vi "Intan_mainControlPanel_64chan_ambulatory_v02.vi"() -> ()   [LabVIEW 2017]
panel:
  in  "Experiment Duration (hr)":u16=20
  out "FileSize(MB)":i16
  out "ADC calib":bool
  in  "Config Hardware Filter":bool=TRUE
  in  "ConfigReg [0:7, aPwr]":bool=TRUE
  in  "R_L source":u8(ring)=1 items=["ON-chip", "OFF-chip"]
  in  "Lower cutoff":u8(ring)=12 items=["10 Hz", "7.5 Hz", "5.0 Hz", "3.0 Hz", "2.5 Hz", "2.0 Hz", "1.5 Hz", "1.0 Hz", "0.75 Hz", "0.5 Hz", "0.3 Hz", "0.25 Hz", "0.10 Hz"]
  in  "Upper cutoff":u8(ring)=12 items=["5.0 kHz", "3.0 kHz", "2.5 kHz", "2.0 kHz", "1.5 kHz", "1.0 kHz", "750 Hz", "500 Hz", "300 Hz", "250 Hz", "200 Hz", "150 Hz", "100 Hz"]
  out "DT stream (us)":dbl
  out "ADC_UART ratio":i16
  in  "UART Stream  Rate (Hz)":u16=20
  out "DT samp (us)":dbl
  out "ADC fs (Hz)":dbl
  in  "Desired Fs (Hz)":u16=100
  in  "Save to SD card":bool=TRUE
  in  "SD File Name Suffix\n (2 digits)":string="51"
  out "Serial Port Type":string
  in  "VISA resource name":refnum<visa-resource-name>="COM33"
  in  "Start Data Stream":bool
  out "HeaderFilePath":path
  in  "Save Display Data":bool
  out "Config Result":string
  out "Teensy response":string
  out "Raw data file path":path
  in  "Save Raw Data":bool
  # "Intan-Teensy Bioelectric Module: \nconfigure hardware and serial port \nAmbulatory 64 chan"
  # "Configure all settings, then click run arrow.\n\nWhen config is complete, click the purple\nbutton to start data stream.\n\nSeparate VI will pop open to display signals"
  # "UART streaming"
  # "TODO 01 May 2017 JE\n\nSTATUS: Operational, beta.\n\nSOFTWARE issues:\n\n - Set decimation ratio to ensure Nsamps in display never exceeds chart limit\nor sensible human visibility bound (for now set chart history length = 50000.\nFor typical max sampling rates of 500 Hz in our applications, this still allows up to 100 s\nof data display (ridiculously long).  In practice, could probably increase performance\nby decreasing chart history to something smaller like 20000.\n\n\n- Make bdf style header and write to file (low priority)\n\n -  Stream to main fig window, Present only does this in subVI (IntanStream_Parallel Loops.vi)\n  SOLN: just pop open subVI automatically when called, but pre-set filters (?)\n\nHARDWARE issues: \n\n\nNeed to gracefully recover when data sync is lost. Option to reboot Teensy and recover connection? \nCurrent error checking not working, don' know why.  Software reset tricky to implement:\nhttps://forum.pjrc.com/archive/index.php/t-24304.html\nBest solution for now, unplug then replug power.  This puts Teensy back into initial state.\n\n-Option to stream subset of channels.  This will allow higher data rate for wireless streaming, if desired."
  # "Intan Amp Config"
  # "Hardware Filter Settings"
  # "ADC Sampling"
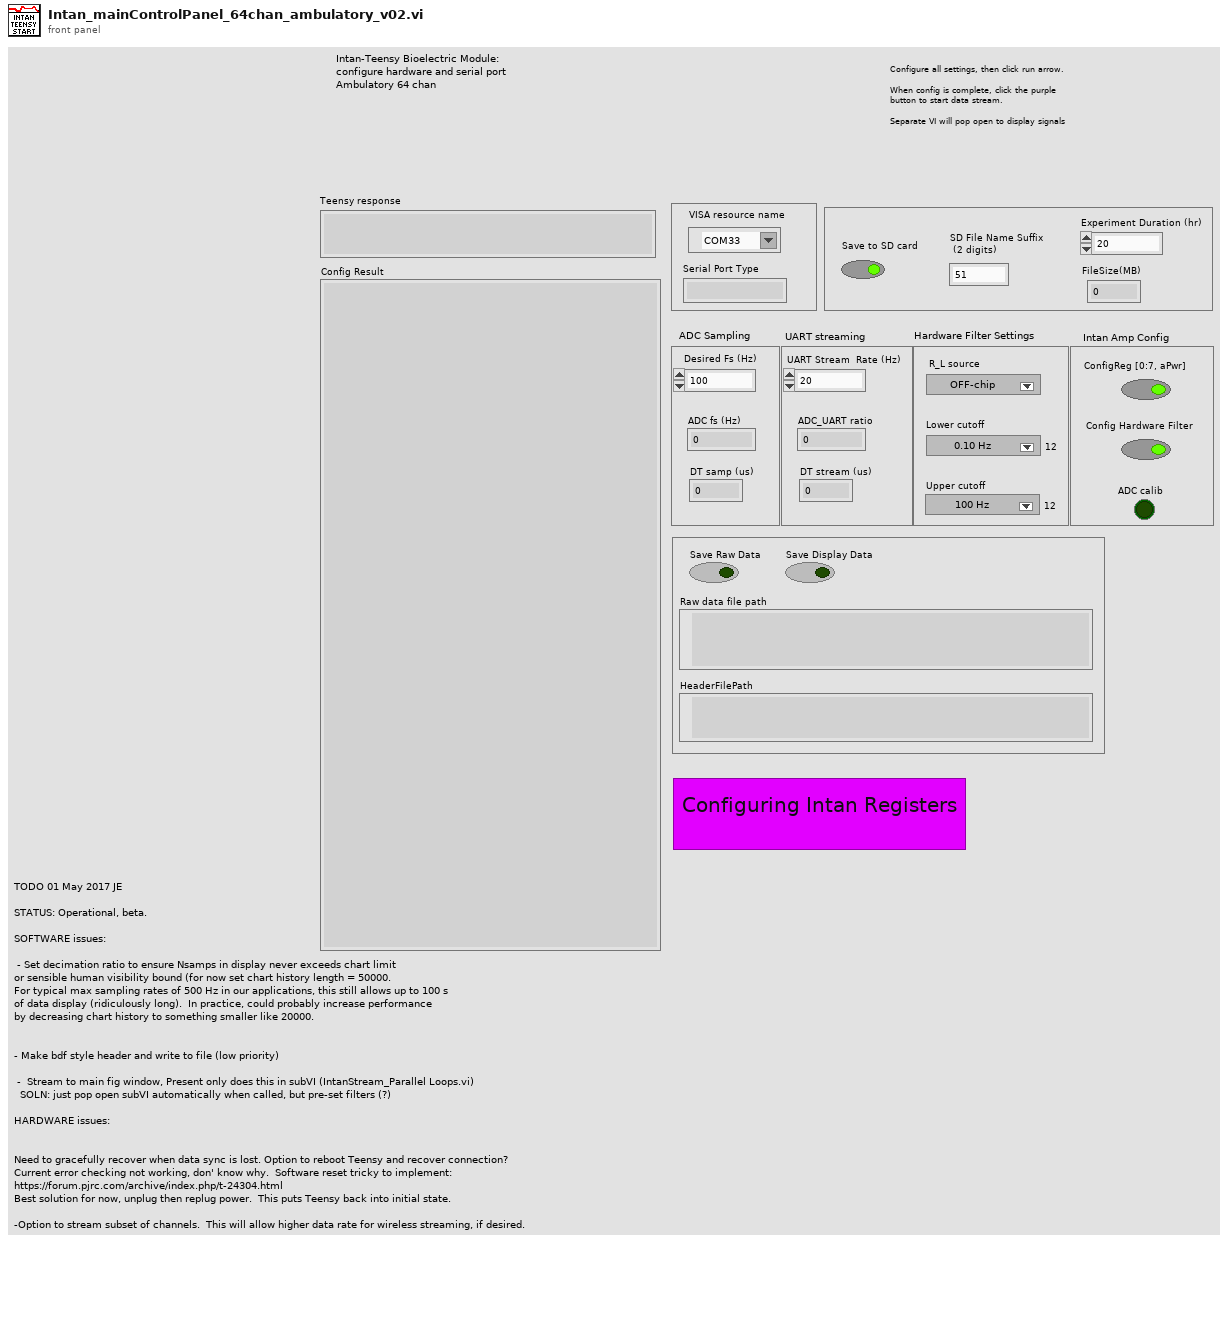
[diagram p1: front panel]
types:
  T1 = enum8{"Enabled", "Disabled", "Disabled and Grayed Out"}
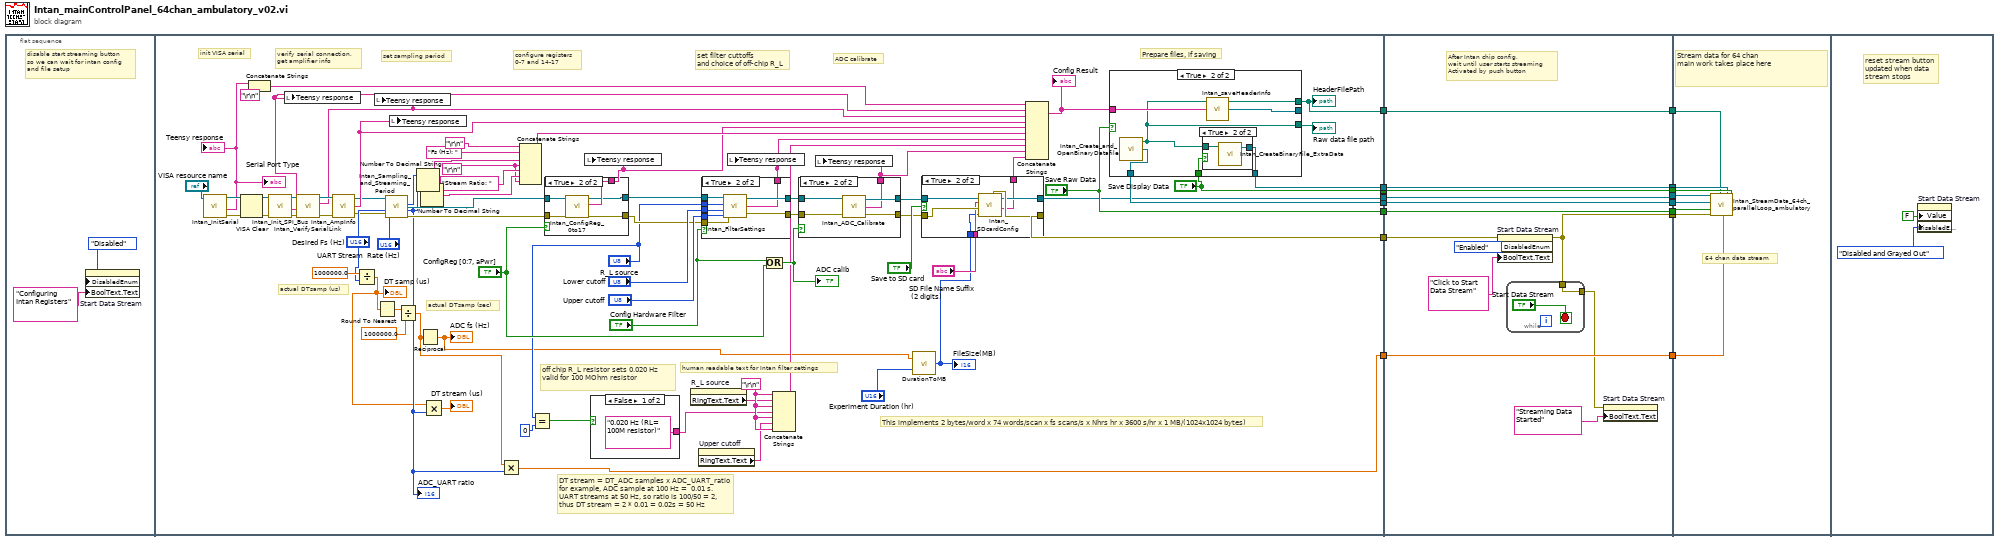
[diagram p0: block diagram]
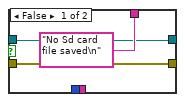
[diagram p2: hidden frame]
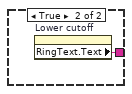
[diagram p3: hidden frame]
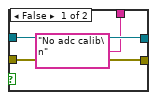
[diagram p4: hidden frame]
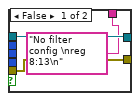
[diagram p5: hidden frame]
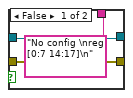
[diagram p6: hidden frame]
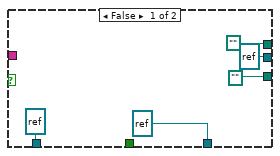
[diagram p7: hidden frame]
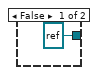
[diagram p8: hidden frame]
diagram:
  n1 = flat-sequence {
    tunnel: [w87] -> w10
    tunnel: [w23] -> w9
    tunnel: [w75] -> w8
    tunnel: ["Save Raw Data"] -> w7
    tunnel: ["Save Display Data"] -> w6
    tunnel: [w35] -> w5
    tunnel: [w57] -> w2
    tunnel: [w33] -> w1
    tunnel: [w153] -> w16
    tunnel: [w159] -> w15
    tunnel: [w158] -> w14
    tunnel: [w157] -> w13
    tunnel: [w156] -> w12
    tunnel: [w155] -> w11
    tunnel: w6 -> [w155]
    tunnel: w7 -> [w156]
    tunnel: w8 -> [w157]
    tunnel: w9 -> [w158]
    tunnel: w10 -> [w159]
    tunnel: w5 -> [w152]
    tunnel: [w151] -> w4
    tunnel: [w150] -> w3
    tunnel: w2 -> [w150]
    tunnel: w1 -> [w151]
    tunnel: w16 -> [w166]
    tunnel: w15 -> [w164]
    tunnel: w14 -> [w169]
    tunnel: w13 -> [w167]
    tunnel: w12 -> [w165]
    tunnel: w11 -> [w168]
    tunnel: w4 -> [w163]
    tunnel: w3 -> [w162]
    frame #0 {
      # "disable start streaming button\nso we can wait for intan config\nand file setup"
      n2 = property on="Start Data Stream" class="Bool (strict)"("DisabledEnum"=T1."Disabled" ("Disabled"), "BoolText.Text"="Configuring Intan Registers" ("Boolean Text.Text")) -> ()  [unwired: 2 in, 2 out]
    }
    frame #1 {
      w52 = "\r\n"
      w26 = "\r\n"
      # "This implements 2 bytes/word x 74 words/scan x fs scans/s x Nhrs hr x 3600 s/hr x 1 MB/(1024x1024 bytes)"
      # "DT stream = DT_ADC samples x ADC_UART_ratio\nfor example, ADC sample at 100 Hz =  0.01 s.\nUART streams at 50 Hz, so ratio is 100/50 = 2,\nthus DT stream = 2 * 0.01 = 0.02s = 50 Hz"
      # "off chip R_L resistor sets 0.020 Hz \nvalid for 100 MOhm resistor"
      # "human readable text for Intan filter settings"
      # "Prepare files, if saving"
      # "ADC calibrate"
      # "set filter cuttoffs \nand choice of off-chip R_L"
      # "configure registers\n0-7 and 14-17"
      # "set sampling period"
      # "verify serial connection,\nget amplifier info"
      # "init VISA serial"
      # "actual DTsamp (sec)"
      # "actual DTsamp (us)"
      n3 = call "Intan_InitSerial.vi"("VISA resource name"="VISA resource name") -> ("VISA resource name out"=w56:refnum<visa-resource-name>, "Text response"=w54:string, "error out"=w86:errorcluster)  [unwired: 3 in]
      "Teensy response" <- w54
      "Serial Port Type" <- w54
      n4 = VISA Clear(VISA resource name=w56, error in (no error)=w86) -> (VISA resource name out=w43:refnum<visa-resource-name>, error out=w42:errorcluster)
      n5 = Concatenate Strings(w54, "\r\n") -> (w39:string)
      n6 = call "Intan_Init_SPI_Bus.vi"("error in"=w42, "VISA resource name"=w43) -> ("error out"=w41:errorcluster, "Text response"=w38:string, "VISA resource name out"=w40:refnum<visa-resource-name>)  [unwired: 3 in]
      n7 = local write "Teensy response"(w38) -> ()
      n8 = call "Intan_VerifySerialLink.vi"("error in"=w41, "VISA resource name"=w40) -> ("error out"=w88:errorcluster, "Text response"=w84:string, "VISA resource name out"=w89:refnum<visa-resource-name>)  [unwired: 7 in]
      n9 = call "Intan_AmpInfo.vi"("error in"=w88, "VISA resource name"=w89) -> ("error out"=w71:errorcluster, "Text response"=w85:string, "VISA resource name out"=w72:refnum<visa-resource-name>)  [unwired: 1 in]
      n10 = Divide(x=1000000.0, y="Desired Fs (Hz)") -> (x/y=w22:dbl)
      "DT samp (us)" <- w22
      n11 = local write "Teensy response"(w84) -> ()
      n12 = Round To Nearest(number=w22) -> (nearest integer value=w78:dbl)
      n13 = call "Intan_Sampling_and_Streaming_Period.vi"("VISA resource name"=w72, "error in"=w71, "Desired Fs (Hz)"="Desired Fs (Hz)", "Desired UART Stream Rate (Hz)"="UART Stream  Rate (Hz)") -> ("VISA resource name out"=w70:refnum<visa-resource-name>, "ADC_UART_Ratio"=w25:i32, "FS actual (Hz)"=w83:i32, "error out"=w69:errorcluster)  [unwired: 1 out]
      "ADC_UART ratio" <- w25
      n14 = local write "Teensy response"(w85) -> ()
      n15 = Divide(x=w78, y=1000000.0 ("x")) -> (x/y=w24:dbl)
      n16 = Number To Decimal String(number=w83) -> (decimal integer string=w82:string)  [unwired: 1 in]
      n17 = Reciprocal(x=w24) -> (1/x=w20:dbl)
      "ADC fs (Hz)" <- w20
      n18 = Number To Decimal String(number=w25) -> (decimal integer string=w27:string)  [unwired: 1 in]
      n19 = Multiply(x=w22, y=w25) -> (x*y=→"DT stream (us)":dbl)
      n20 = Multiply(x=w24, y=w25) -> (x*y=w23:dbl)
      n21 = Concatenate Strings("\r\n", "Fs (Hz): " ("string"), w82, w26, "Stream Ratio: " ("string"), w27, w26) -> (w81:string)
      n22 = Equal?(x="R_L source", y=u8 0) -> (x = y?=w47:bool)
      n23 = case shown="True" "ConfigReg [0:7, aPwr]" {
        tunnel: w70 -> [w125 w131]
        tunnel: w69 -> [w124 w130]
        tunnel: ["No config \nreg [0:7 14:17]\n" ("Text response") w129] -> w68
        tunnel: [w125 w128] -> w65
        tunnel: [w124 w127] -> w64
        frame False {
        }
        frame True {
          n24 = call "Intan_ConfigReg_0to17.vi"("error in"=w130, "VISA resource name"=w131) -> ("error out"=w127:errorcluster, "Text response"=w129:string, "VISA resource name out"=w128:refnum<visa-resource-name>)  [unwired: 7 in]
        }
      }
      n25 = local write "Teensy response"(w68) -> ()
      n26 = case shown="False" w47 {
        tunnel: ["0.020 Hz (RL= 100M resistor)" ("string") w104] -> w45
        frame False {
        }
        frame True {
          n27 = property on="Lower cutoff" class="Ring (strict)"() -> ("RingText.Text"=w104:string)  [unwired: 2 in, 2 out]
        }
      }
      n28 = property on="R_L source" class="Ring (strict)"() -> ("RingText.Text"=w50:string)  [unwired: 2 in, 2 out]
      n29 = property on="Upper cutoff" class="Ring (strict)"() -> ("RingText.Text"=w51:string)  [unwired: 2 in, 2 out]
      n30 = case shown="True" "Config Hardware Filter" {
        tunnel: "R_L source" -> [_ w123]
        tunnel: "Lower cutoff" -> [_ w122]
        tunnel: "Upper cutoff" -> [_ w121]
        tunnel: w65 -> [w115 w120]
        tunnel: w64 -> [w114 w119]
        tunnel: [w115 w118] -> w63
        tunnel: [w114 w117] -> w62
        tunnel: ["No filter config \nreg 8:13\n" ("Text response") w116] -> w61
        frame False {
        }
        frame True {
          n31 = call "Intan_FilterSettings.vi"("VISA resource name"=w120, "R_L source"=w123, "Lower cutoff"=w122, "Upper cutoff"=w121, "error in"=w119) -> ("VISA resource name out"=w118:refnum<visa-resource-name>, "Text response"=w116:string, "error out"=w117:errorcluster)
        }
      }
      n32 = local write "Teensy response"(w61) -> ()
      n33 = Or(x="Config Hardware Filter", y="ConfigReg [0:7, aPwr]") -> (x .or. y?=w60:bool)
      "ADC calib" <- w60
      n34 = Concatenate Strings(w52, w50, w52, w45, w52, w51, w52) -> (w48:string)
      n35 = case shown="True" w60 {
        tunnel: w63 -> [w107 w112]
        tunnel: w62 -> [w106 w111]
        tunnel: [w106 w110] -> w34
        tunnel: [w107 w109] -> w32
        tunnel: ["No adc calib\n" ("Text response") w108] -> w49
        frame False {
        }
        frame True {
          n36 = call "Intan_ADC_Calibrate.vi"("error in"=w111, "VISA resource name"=w112) -> ("error out"=w110:errorcluster, "Text response"=w108:string, "VISA resource name out"=w109:refnum<visa-resource-name>)  [unwired: 1 in]
        }
      }
      n37 = local write "Teensy response"(w49) -> ()
      n38 = call "DurationToMB.vi"("Experiment Duration (hr)"="Experiment Duration (hr)", "fs (hz)"=w20) -> ("FileSize(MB)"=w21:i16)
      "FileSize(MB)" <- w21
      n39 = case shown="True" "Save to SD card" {
        tunnel: ["No Sd card file saved\n" ("Text response") w96] -> w36
        tunnel: [w93 w102] -> w35
        tunnel: w34 -> [w93 w101]
        tunnel: w32 -> [w94 w100]
        tunnel: [w94 w99] -> w33
        tunnel: "SD File Name Suffix\n (2 digits)" -> [_ w98]
        tunnel: w21 -> [_ w97]
        frame False {
        }
        frame True {
          n40 = call "Intan_SDcardConfig.vi"("VISA resource name"=w100, "SdFilename"=w98, "error in"=w101, "FileSize(MB)"=w97) -> ("error out"=w102:errorcluster, "VISA resource name out"=w99:refnum<visa-resource-name>, "SDCardResultStr"=w96:string)  [unwired: 3 out]
        }
      }
      n41 = Concatenate Strings(w39, w38, w84, w85, w68, w81, w61, w48, w49, w36) -> (w76:string)
      "Config Result" <- w76
      n42 = case shown="True" "Save Raw Data" {
        tunnel: [refnum<file> refnum ("refnum out") w143] -> w87
        tunnel: w76 -> [_ w142]
        tunnel: [refnum<file> refnum ("refnum out") w141] -> w75
        tunnel: "Save Display Data" -> [_ w140]
        tunnel: [path "" w139] -> w57
        tunnel: [path "" w138] -> w66
        tunnel: [refnum<file> refnum ("hdr_file_ref_num_out") w137] -> _
        frame False {
        }
        frame True {
          n43 = call "Intan_Create_and_OpenBinaryDatafile.vi"() -> ("file path"=w138:path, "refnum out"=w143:refnum<file>)  [unwired: 2 in, 1 out]
          n44 = case shown="True" w140 {
            tunnel: w138 -> [_ w146]
            tunnel: [refnum<file> refnum ("refnum out") w145] -> w141
            frame False {
            }
            frame True {
              n45 = call "Intan_CreateBinaryFile_ExtraData.vi"("DataFilePath"=w146) -> ("refnum out"=w145:refnum<file>)  [unwired: 3 in, 1 out]
            }
          }
          n46 = call "Intan_saveHeaderInfo.vi"("header text"=w142, "DataFilePath"=w138) -> ("hdr_file_ref_num_out"=w137:refnum<file>, "HeaderFilePath"=w139:path)  [unwired: 1 in, 1 out]
        }
      }
      "HeaderFilePath" <- w57
      "Raw data file path" <- w66
    }
    frame #2 {
      # "After Intan chip config,\nwait until user starts streaming\nActivated by push button"
      n47 = property on="Start Data Stream" class="Bool (strict)"(error in=w152, "DisabledEnum"=T1."Enabled" ("Disabled"), "BoolText.Text"="Click to Start Data Stream" ("Boolean Text.Text")) -> (error out=w153:errorcluster)  [unwired: 1 in, 1 out]
      n48 = while {
        tunnel: w153 -> [w160]
        tunnel: [w160] -> w148
        stop <- "Start Data Stream" stop-if-true
      }
      n49 = property on="Start Data Stream" class="Bool (strict)"(error in=w148, "BoolText.Text"="Streaming Data Started" ("Boolean Text.Text")) -> ()  [unwired: 1 in, 2 out]
    }
    frame #3 {
      # "64 chan data stream"
      # "Stream data for 64 chan\nmain work takes place here"
      n50 = call "Intan_StreamData_64ch_parallelLoop_ambulatory.vi"("VISA resource name"=w163, "refnum in"=w164, "Save Binary Data"=w165, "error in"=w166, "hdr fpath"=w162, "DT_scale (sec)"=w169, "aux file ref num"=w167, "save aux file"=w168) -> ()  [unwired: 8 in, 4 out]
    }
    frame #4 {
      # "reset stream button \nupdated when data\nstream stops"
      n51 = property on="Start Data Stream" class="Bool (strict)"("Value"=FALSE ("Start Data Stream"), "DisabledEnum"=T1."Disabled and Grayed Out" ("Disabled")) -> ()  [unwired: 2 in, 2 out]
    }
  }
